vi "lv-ros-bridge_READ.vi"(8 "error in (no error)":errorcluster, 9 "Topic to subscribe":string="/", 10 "rosbridge port":u16=9090, 11 "rosbridge server IP":string="192.168.164.128") -> (0 "error out":errorcluster)   [LabVIEW 2015]
uses:
  <vilib>/Intelligent Energy/WebSockets API/WebSockets/WebSockets.lvlib
panel:
  out "value":T1
  in  "szablon":T1
  out "Opcode":u8
  out "Data":string
  in  "stop":bool
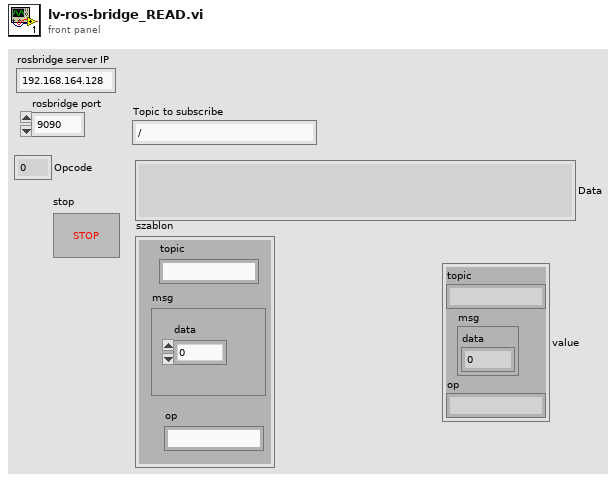
[diagram p1: front panel]
types:
  T1 = cluster{"topic":string, "msg":cluster{"data":i16}, "op":string}
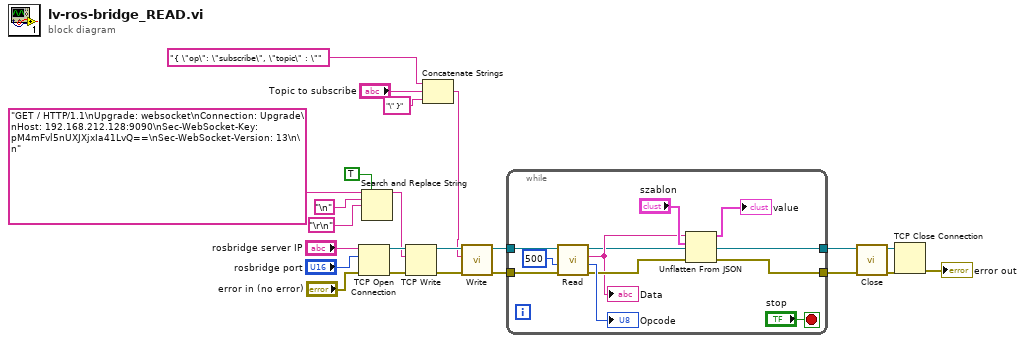
[diagram p0: block diagram]
diagram:
  n1 = TCP Open Connection(address="rosbridge server IP", remote port or service name="rosbridge port", error in (no error)="error in (no error)") -> (connection ID=w21:refnum<k5>, error out=w20:errorcluster)  [unwired: 2 in]
  n2 = Search and Replace String(replace all?=TRUE ("replace all? (F)"), input string="GET / HTTP/1.1\nUpgrade: websocket\nConnection: Upgrade\nHost: 192.168.212.128:9090\nSec-WebSocket-Key: pM4mFvl5nUXJXjxIa41LvQ==\nSec-WebSocket-Version: 13\n\n", search string="\n", replace string="\r\n") -> (result string=w5:string)  [unwired: 4 in, 3 out]
  n3 = TCP Write(connection ID=w21, data in=w5, error in (no error)=w20) -> (connection ID out=w17:refnum<k5>, error out=w16:errorcluster)  [unwired: 1 in, 1 out]
  n4 = Concatenate Strings("{ \"op\": \"subscribe\", \"topic\" : \"", "Topic to subscribe", "\" }") -> (w3:string)
  n5 = call <vilib>:"Write.vi"("error in (no error)"=w16, "Data"=w3, "WebSocket Connection in"=w17) -> ("error out"=w12:errorcluster, "WebSocket Connection out"=w13:refnum<k5>)  [unwired: 7 in]
  n6 = while {
    tunnel: [w25] -> w15
    tunnel: [w24] -> w14
    tunnel: w13 -> [w34]
    tunnel: w12 -> [w33]
    stop <- "stop" stop-if-true
    n7 = call <vilib>:"Read.vi"("error in (no error)"=w33, "timeout ms (5000)"=500, "WebSocket Connection in"=w34) -> ("error out"=w28:errorcluster, "Opcode"=→"Opcode":u8, "Data"=w27:string, "WebSocket Connection out"=w25:refnum<k5>)  [unwired: 5 in]
    "Data" <- w27
    n8 = Unflatten From JSON(JSON string=w27, type and defaults="szablon", error in (no error)=w28) -> (value=→"value":T1, error out=w24:errorcluster)  [unwired: 4 in]
  }
  n9 = call <vilib>:"Close.vi"("error in (no error)"=w14, "WebSocket Connection in"=w15) -> ("error out"=w18:errorcluster, "WebSocket Connection in"=w19:refnum<k5>)  [unwired: 8 in]
  n10 = TCP Close Connection(connection ID=w19, error in (no error)=w18) -> (error out=→"error out":errorcluster)  [unwired: 1 in, 1 out]
